vi "auto_ir_config.vi"() -> ()   [LabVIEW 2012, in "BlockParty4150.lvrbt"]
uses:
  BlockParty4150.lvrbt
  <vilib>/NXT/Subs/LVHSConnector.ctl
  <vilib>/NXT/LegoClasses/BrickReference/BrickReference.lvclass
  <vilib>/NXT/Block Support/NXT_ButtonSelector.ctl
  <vilib>/NXT/HiTechnic/HiTechnic Controls/HiTechnic Port.ctl
  <vilib>/NXT/Block Support/NXT_InputPort.ctl
  <vilib>/NXT/Hardware/Plugins/Tetrix DC Motor/TetrixDCMotorAddress.ctl
  <vilib>/NXT/Dual Mode Library/Display/drawText.vi
  <vilib>/NXT/Dual Mode Library/Waits/Wait_Num(msec).vi
  <vilib>/NXT/Dual Mode Library/prims/inRangeAndCoerce/inRangeAndCoerce_int.vi
  <vilib>/NXT/Dual Mode Library/Display/drawNumber.vi
  <vilib>/NXT/Dual Mode Library/Sound/Tone.vi
  <vilib>/NXT/NXTIO Xnodes/NXTIONodeSubVIs/TETRIX IO Move DC Motors.vi
  <vilib>/NXT/NXTIO Xnodes/NXTIONodeSubVIs/TETRIX IO Stop DC Motors.vi
  <vilib>/NXT/NXTIO Xnodes/AddressXNode/NXTIOAddress.xnode
  <vilib>/NXT/NXTIO Xnodes/NXTIOXNode/NXTIO.xnode
panel:
  out "Enabled":bool
  out "iter":i32
  out "NXT":T1
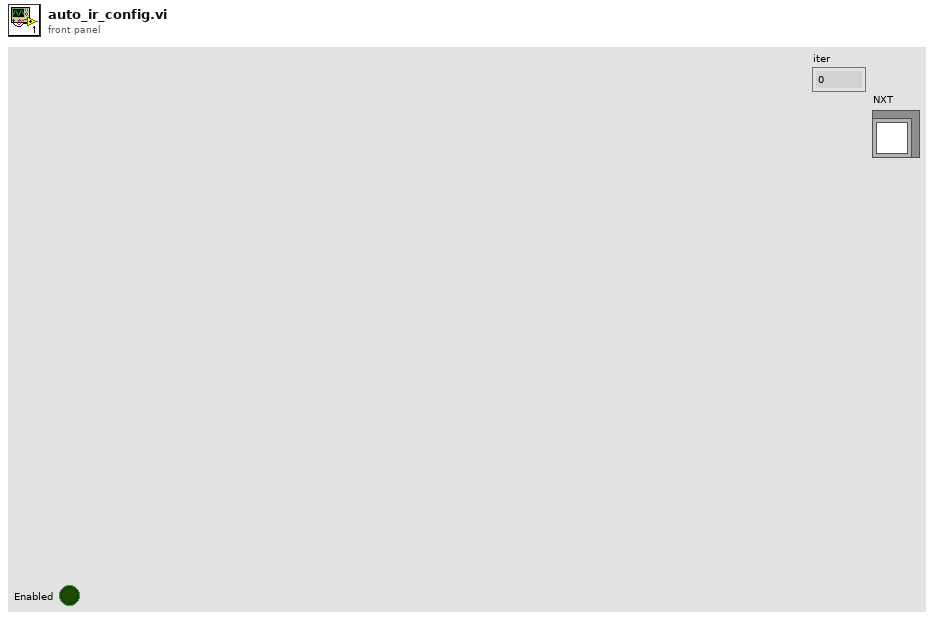
[diagram p1: front panel]
types:
  T1 = typedef "LVHSConnector.ctl" = refnum<class "BrickReference.lvclass">
  T2 = typedef "NXT_ButtonSelector.ctl" = u16
  T3 = typedef "TetrixDCMotorAddress.ctl" = i16
  T4 = typedef "HiTechnic Port.ctl" = cluster{"Port":T5, "MUX Port":u8}
  T5 = typedef "NXT_InputPort.ctl" = u8
  T6 = cluster{"Direction (0-9)":i16, "Signal Strength (Array)":u8[]}
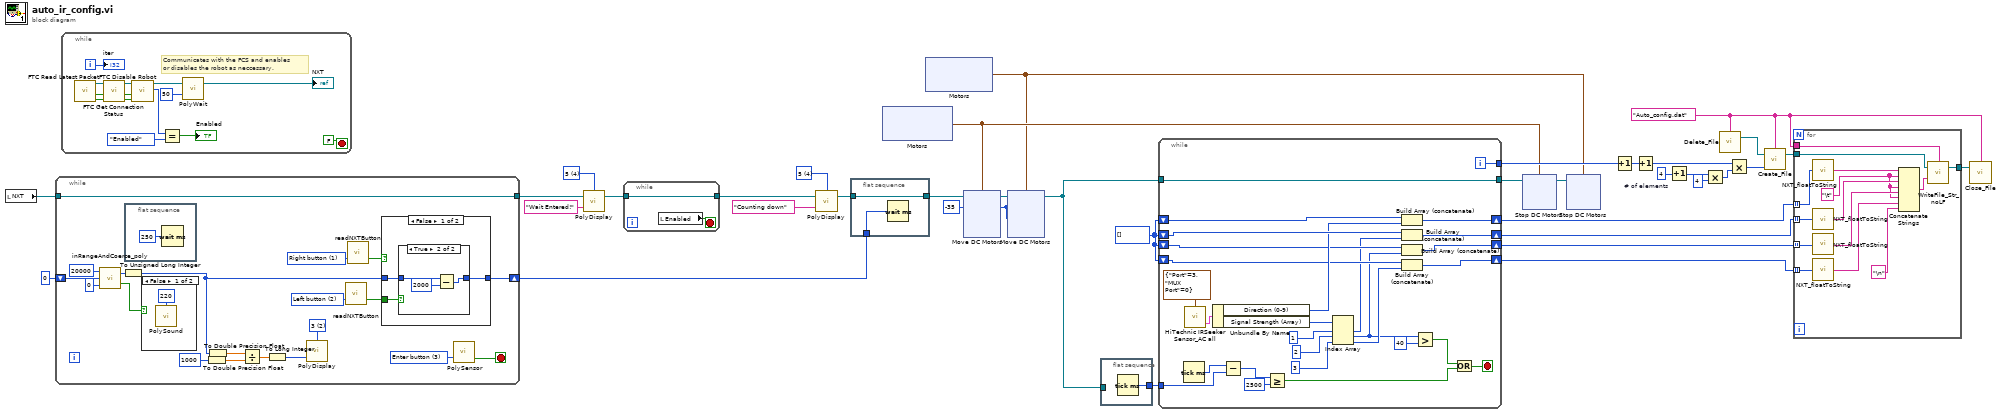
[diagram p0: block diagram]
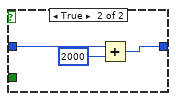
[diagram p4: hidden frame]
diagram:
  w6 = i8 -35 ("Power/Speed 1")
  w14 = i16 4 items=["1", "2", "3", "4", "5", "6", "7", "8"] ("Line")
  w15 = i16 4 items=["1", "2", "3", "4", "5", "6", "7", "8"] ("Line")
  w22 = u32[] []
  w31 = 4  # # of elements
  w27 = "Auto_config.dat" ("Filename")
  n1 = local read "NXT"() -> (w9:T1)
  n2 = while {
    tunnel: [w57] -> w17
    tunnel: w9 -> [w57]
    shift-right: [w50] -> w18
    shift-left: u32 0 ("Power/Speed 1") -> [w43]
    stop <- w55 stop-if-true
    w49 = i16 2 items=["1", "2", "3", "4", "5", "6", "7", "8"] ("Line")
    w52 = T2 1 items=["Enter button"=3, "Left button"=2, "Right button"=1] ("Button (Enter button)")
    w51 = T2 2 items=["Enter button"=3, "Left button"=2, "Right button"=1] ("Button (Enter button)")
    w56 = T2 3 items=["Enter button"=3, "Left button"=2, "Right button"=1] ("Button (Enter button)")
    n3 = call-poly <vilib>:"inRangeAndCoerce_poly.vi"("lower limit"=0, "x"=w43, "upper limit"=20000) -> ("In Range?"=w38:bool, "coerced(x)"=w40:i32)
    n4 = To Unsigned Long Integer(number=w40) -> (unsigned 32bit integer=w39:u32)
    n5 = flat-sequence {
      frame #0 {
        n6 = Wait (ms)(milliseconds to wait=u32 250) -> ()  [unwired: 1 out]
      }
    }
    n7 = case shown="False" w38 {
      frame False {
        n8 = call-poly <vilib>:"PolySound.vi"("Tone (440 Hz)"=u16 220) -> ()  [unwired: 3 in, 1 out]
      }
      frame True {
      }
    }
    n9 = To Double Precision Float(number=u32 1000 ("Power/Speed 1")) -> (double precision float=w44:dbl)
    n10 = To Double Precision Float(number=w39) -> (double precision float=w46:dbl)
    n11 = Divide(x=w46, y=w44) -> (x/y=w47:dbl)
    n12 = To Long Integer(number=w47) -> (32bit integer=w45:i32)
    n13 = call-poly <vilib>:"PolyDisplay.vi"("number"=w45, "Line"=w49) -> ()  [unwired: 2 in, 1 out]
    n14 = call <vilib>:"readNXTButton.vi"("Button (Enter button)"=w51) -> ("Yes/No"=w54:bool)  [unwired: 2 in, 1 out]
    n15 = call <vilib>:"readNXTButton.vi"("Button (Enter button)"=w52) -> ("Yes/No"=w53:bool)  [unwired: 2 in, 1 out]
    n16 = case shown="False" w53 {
      tunnel: w54 -> [w62 _]
      tunnel: [w61 w68] -> w50
      tunnel: w39 -> [w60 w69]
      frame False {
        n17 = case shown="True" w62 {
          tunnel: [w63 w65] -> w61
          tunnel: w60 -> [w63 w66]
          frame False {
          }
          frame True {
            n18 = Subtract(x=w66, y=u32 2000) -> (x-y=w65:u32)
          }
        }
      }
      frame True {
        n19 = Add(x=w69, y=u32 2000) -> (x+y=w68:u32)
      }
    }
    n20 = call-poly <vilib>:"PolySensor.vi"("Button (Enter button)"=w56) -> ("Yes/No"=w55:bool)  [unwired: 2 in, 1 out]
  }
  n21 = while {
    i -> [w71]
    stop <- FALSE stop-if-true
    # "Communicates with the FCS and enables \nor disables the robot as neccessary."
    n22 = call <vilib>:"FTC Read Latest Packet.vi"() -> ("Packet Received?"=w81:bool, "Stopped?"=w80:bool, "NXT"=w83:T1)  [unwired: 6 in, 3 out]
    n23 = call <vilib>:"FTC Get Connection Status.vi"("Packet Received?"=w81, "Stopped?"=w80, "NXT"=w83) -> ("Online?"=w73:bool, "Stopped?"=w74:bool, "NXT"=w82:T1)  [unwired: 5 in]
    n24 = call <vilib>:"FTC Disable Robot.vi"("Online?"=w73, "Stopped?"=w74, "NXT"=w82) -> ("Enabled?"=w77:enum16{"Disabled", "Enabled"}, "NXT"=w79:T1)  [unwired: 3 in]
    n25 = Equal?(x=w77, y=enum16{"Disabled", "Enabled"}."Enabled") -> (x = y?=→"Enabled":bool)
    n26 = call-poly <vilib>:"PolyWait.vi"("Time (100 msec)"=u32 50 ("Time (msec)"), "NXT"=w79) -> ("NXT"=→"NXT":T1)  [unwired: 2 in]
    "iter" <- w71
  }
  n27 = call-poly <vilib>:"PolyDisplay.vi"("Text"="Wait Entered!", "NXT"=w17, "Line"=w15) -> ("NXT"=w11:T1)  [unwired: 1 in]
  n28 = while {
    tunnel: [w84] -> w10
    tunnel: w11 -> [w84]
    stop <- w85 stop-if-true
    n29 = local read "Enabled"() -> (w85:bool)
  }
  n30 = call-poly <vilib>:"PolyDisplay.vi"("Text"="Counting down", "NXT"=w10, "Line"=w14) -> ("NXT"=w12:T1)  [unwired: 1 in]
  n31 = flat-sequence {
    tunnel: w12 -> [w87]
    tunnel: [w87] -> w8
    tunnel: w18 -> [w86]
    frame #0 {
      n32 = Wait (ms)(milliseconds to wait=w86) -> ()  [unwired: 1 out]
    }
  }
  n33 = xnode "Motors"() -> ("Motor"=w3:cluster{"TetrixDCMotor":T3, "TetrixDCMotor":T3})
  n34 = xnode "Motors"() -> ("Motor"=w2:cluster{"TetrixDCMotor":T3, "TetrixDCMotor":T3})
  n35 = xnode "Move DC Motors"("Power/Speed 2"=w6, "Power/Speed 1"=w6, "Motors"=w3, "NXT"=w8) -> ("NXT"=w7:T1)
  n36 = xnode "Move DC Motors"("Power/Speed 2"=w6, "Power/Speed 1"=w6, "Motors"=w2, "NXT"=w7) -> ("NXT"=w1:T1)
  n37 = flat-sequence {
    tunnel: [w88] -> w37
    tunnel: w1 -> [_]
    frame #0 {
      n38 = Tick Count (ms)() -> (millisecond timer value=w88:u32)
    }
  }
  n39 = while {
    tunnel: w37 -> [w115]
    tunnel: [w113] -> w29
    shift-right: [w112] -> w25
    shift-left: w22 -> [w111]
    shift-right: [w108] -> w24
    shift-left: w22 -> [w109]
    shift-right: [w97] -> w21
    shift-left: w22 -> [w100]
    shift-right: [w96] -> w20
    shift-left: w22 -> [w99]
    tunnel: w1 -> [w95]
    tunnel: [w95] -> w5
    i -> [w113]
    stop <- w92 stop-if-true
    n40 = Tick Count (ms)() -> (millisecond timer value=w116:u32)
    n41 = call <vilib>:"HiTechnic IRSeeker Sensor_AC all.vi"("Port/MUX"=T4 {"Port"=3, "MUX Port"=0}) -> ("All Info"=w107:T6)  [unwired: 2 in, 1 out]
    n42 = Unbundle By Name(w107) -> ("Direction (0-9)"=w103:i16, "Signal Strength (Array)"=w106:u8[])
    n43 = Subtract(x=w116, y=w115) -> (x-y=w110:u32)
    n44 = Greater Or Equal?(x=w110, y=u32 2500) -> (x >= y?=w90:bool)
    n45 = Index Array(array=w106, index #1=1 ("index"), index #2=2 ("index"), index #3=3 ("index")) -> (element #1=w94:u8, element #2=w89:u8, element #3=w98:u8)
    n46 = Build Array (concatenate)(w111, w103) -> (w112:u32[])
    n47 = Build Array (concatenate)(w109, w94) -> (w108:u32[])
    n48 = Build Array (concatenate)(w100, w89) -> (w97:u32[])
    n49 = Build Array (concatenate)(w99, w98) -> (w96:u32[])
    n50 = Greater?(x=w89, y=u8 40) -> (0:w91:bool)
    n51 = Or(x=w91, y=w90) -> (x .or. y?=w92:bool)
  }
  n52 = xnode "Stop DC Motors"("Motors"=w3, "NXT"=w5) -> ("NXT"=w4:T1)
  n53 = xnode "Stop DC Motors"("Motors"=w2, "NXT"=w4) -> ()  [unwired: 1 out]
  n54 = Increment(x=w29) -> (x+1=w28:i32)
  n55 = Increment(x=w28) -> (x+1=w35:i32)
  n56 = Increment(x=w31) -> (x+1=w32:i32)
  n57 = Multiply(x=w32, y=u32 4) -> (x*y=w33:u32)
  n58 = call <vilib>:"Delete_File.vi"("Filename"=w27) -> ("NXT"=w36:T1)  [unwired: 3 in]
  n59 = Multiply(x=w35, y=w33) -> (x*y=w23:u32)
  n60 = call <vilib>:"Create_File.vi"("File Size (256)"=w23, "NXT"=w36, "Filename"=w27) -> ("NXT"=w26:T1)  [unwired: 1 out]
  n61 = for {
    tunnel: w27 -> [w130]
    tunnel: w26 -> [w129]
    tunnel: [w128] -> w30
    tunnel: w25 -> [w127] mode=indexing
    tunnel: w24 -> [w125] mode=indexing
    tunnel: w21 -> [w118] mode=indexing
    tunnel: w20 -> [w117] mode=indexing
    w121 = "\t" ("string")
    n62 = call <vilib>:"NXT_floatToString.vi"("number"=w127) -> ("string"=w124:string)
    n63 = call <vilib>:"NXT_floatToString.vi"("number"=w125) -> ("string"=w123:string)
    n64 = call <vilib>:"NXT_floatToString.vi"("number"=w118) -> ("string"=w122:string)
    n65 = call <vilib>:"NXT_floatToString.vi"("number"=w117) -> ("string"=w120:string)
    n66 = Concatenate Strings(w124, w121, w123, w121, w122, w121, w120, "\n") -> (w126:string)
    n67 = call <vilib>:"WriteFile_Str_noLF.vi"("String"=w126, "NXT"=w129, "Filename"=w130) -> ("NXT"=w128:T1)  [unwired: 1 in]
  }
  n68 = call <vilib>:"Close_File.vi"("NXT"=w30, "Filename"=w27) -> ()  [unwired: 2 in, 1 out]
